vi "VI Anlagengrenzwerte.vi"() -> ()   [LabVIEW 2020, in "Anlagengrenzwerte.lvlib"]
uses:
  Seiten/Anlagengrenzwerte/Anlagengrenzwerte.lvlib
  Visualisierungs Elemente/Button.ctl
  Seiten/Anlagengrenzwerte/Anlagen-Grenzwerte Anzeige.ctl
  Seiten/Anlagengrenzwerte/Anlagen-Parameter Anzeige.ctl
  Seiten/Anlagengrenzwerte/FGV Anlagengrenzwerte Aktionen.ctl
  Seiten/Anlagenuebersicht/Aktionen Ausgabefaelder einfaerben.ctl
  Passwortverwaltung/FGV Passwort Aktion.ctl
  Allgemein/Aktionen Daten am cRIO speichern.ctl
  Seiten/FT-IR/FGV FT-IR Diagnose Aktionen.ctl
  Status Analysatoren/Aktion Status Analysatoren.ctl
  Status Analysatoren/Status Analysatoren.lvlib
  Passwortverwaltung/Passwort.lvlib
  Allgemein/allgemeine Sub-VIs.lvlib
  Seiten/Anlagenuebersicht/VisBx Anzeige/Anlagenuebersicht.lvlib
  Seiten/FT-IR/FT-IR.lvlib
  cRIO/PC/Kommunikation mit cRIO.lvlib
  Visualisierungs Elemente/Zahlen-Eingabefeld.ctl
panel:
  out "HL zu FT-IR:":sgl caption="°C" format="%.1f"
  out "Durchfluss CalGas:":sgl caption="l/min" format="%.1f"
  out "Schaltschranktemperatur:":sgl caption="°C" format="%.1f"
  out "Gaskühler:":sgl caption="°C" format="%.1f"
  out "Heizung FT-IR Messzelle:":sgl caption="°C" format="%.1f"
  out "Heizung Extern SP2:":sgl caption="°C" format="%.1f"
  out "Heizung Extern SP1:":sgl caption="°C" format="%.1f"
  out "Heizung Pumpe:":sgl caption="°C" format="%.1f"
  out "Heizung Filter:":sgl caption="°C" format="%.1f"
  out "Druck Kalter Block:":sgl caption="mbar" format="%.1f"
  out "Druck Ausgang:":sgl caption="mbar"
  out "Durchfluss FT-IR:":sgl caption="l/min" format="%.1f"
  out "Eingangsdruck":sgl caption="atm" format="%.3f"
  in  "speichern":T1
  in  "Anlagen-Grenzwerte":T2 {"Heizleitung zu FT-IR:"."Abschalt-Max" format="%#_5g"; "Heizleitung zu FT-IR:"."Abschalt-Min" format="%#_5g"; "Heizleitung zu FT-IR:"."Warn-Max" format="%#_5g"; "Heizleitung zu FT-IR:"."Warn-Min" format="%#_5g"; "Heizleitung zu FT-IR:"."Sollwert" format="%#_5g"; "Heizleitung zu FT-IR:"."Regler" items=["inaktiv", "aktiv"]; "Druck Kalter Block:"."Abschalt-Max" format="%#_5g"; "Druck Kalter Block:"."Abschalt-Min" format="%#_5g"; "Druck Kalter Block:"."Warn-Max" format="%#_5g"; "Druck Kalter Block:"."Warn-Min" format="%#_5g"; "Druck Kalter Block:"."Sollwert" format="%#_5g"; "Druck Kalter Block:"."Regler" items=["inaktiv", "aktiv"]; "Durchfluss CalGas:"."Abschalt-Max" format="%#_5g"; "Durchfluss CalGas:"."Abschalt-Min" format="%#_5g"; "Durchfluss CalGas:"."Warn-Max" format="%#_5g"; "Durchfluss CalGas:"."Warn-Min" format="%#_5g"; "Durchfluss CalGas:"."Sollwert" format="%#_5g"; "Durchfluss CalGas:"."Regler" items=["inaktiv", "aktiv"]; "Heizleitung Extern SP2:"."Abschalt-Max" format="%#_5g"; "Heizleitung Extern SP2:"."Abschalt-Min" format="%#_5g"; "Heizleitung Extern SP2:"."Warn-Max" format="%#_5g"; "Heizleitung Extern SP2:"."Warn-Min" format="%#_5g"; "Heizleitung Extern SP2:"."Sollwert" format="%#_5g"; "Heizleitung Extern SP2:"."Regler" items=["inaktiv", "aktiv"]; "Gaskühler:"."Abschalt-Max" format="%#_5g"; "Gaskühler:"."Abschalt-Min" format="%#_5g"; "Gaskühler:"."Warn-Max" format="%#_5g"; "Gaskühler:"."Warn-Min" format="%#_5g"; "Gaskühler:"."Sollwert" format="%#_5g"; "Gaskühler:"."Regler" items=["inaktiv", "aktiv"]; "Heizleitung Extern SP1:"."Abschalt-Max" format="%#_5g"; "Heizleitung Extern SP1:"."Abschalt-Min" format="%#_5g"; "Heizleitung Extern SP1:"."Warn-Max" format="%#_5g"; "Heizleitung Extern SP1:"."Warn-Min" format="%#_5g"; "Heizleitung Extern SP1:"."Sollwert" format="%#_5g"; "Heizleitung Extern SP1:"."Regler" items=["inaktiv", "aktiv"]; "Schaltschranktemperatur:"."Abschalt-Max" format="%#_5g"; "Schaltschranktemperatur:"."Abschalt-Min" format="%#_5g"; "Schaltschranktemperatur:"."Warn-Max" format="%#_5g"; "Schaltschranktemperatur:"."Warn-Min" format="%#_5g"; "Schaltschranktemperatur:"."Sollwert" format="%#_5g"; "Schaltschranktemperatur:"."Regler" items=["inaktiv", "aktiv"]; "FT-IR Heizung Messzelle:"."Abschalt-Max" format="%#_5g"; "FT-IR Heizung Messzelle:"."Abschalt-Min" format="%#_5g"; "FT-IR Heizung Messzelle:"."Warn-Max" format="%#_5g"; "FT-IR Heizung Messzelle:"."Warn-Min" format="%#_5g"; "FT-IR Heizung Messzelle:"."Sollwert" format="%#_5g"; "FT-IR Heizung Messzelle:"."Regler" items=["inaktiv", "aktiv"]; "Heizung Pumpe:"."Abschalt-Max" format="%#_5g"; "Heizung Pumpe:"."Abschalt-Min" format="%#_5g"; "Heizung Pumpe:"."Warn-Max" format="%#_5g"; "Heizung Pumpe:"."Warn-Min" format="%#_5g"; "Heizung Pumpe:"."Sollwert" format="%#_5g"; "Heizung Pumpe:"."Regler" items=["inaktiv", "aktiv"]; "Heizung Filterblock:"."Abschalt-Max" format="%#_5g"; "Heizung Filterblock:"."Abschalt-Min" format="%#_5g"; "Heizung Filterblock:"."Warn-Max" format="%#_5g"; "Heizung Filterblock:"."Warn-Min" format="%#_5g"; "Heizung Filterblock:"."Sollwert" format="%#_5g"; "Heizung Filterblock:"."Regler" items=["inaktiv", "aktiv"]; "Heizleitungen intern:"."Abschalt-Max" format="%#_5g"; "Heizleitungen intern:"."Abschalt-Min" format="%#_5g"; "Heizleitungen intern:"."Warn-Max" format="%#_5g"; "Heizleitungen intern:"."Warn-Min" format="%#_5g"; "Heizleitungen intern:"."Sollwert" format="%#_5g"; "Heizleitungen intern:"."Regler" items=["inaktiv", "aktiv"]; "Druck Ausgang:"."Abschalt-Max" format="%#_5g"; "Druck Ausgang:"."Abschalt-Min" format="%#_5g"; "Druck Ausgang:"."Warn-Max" format="%#_5g"; "Druck Ausgang:"."Warn-Min" format="%#_5g"; "Druck Ausgang:"."Sollwert" format="%#_5g"; "Druck Ausgang:"."Regler" items=["inaktiv", "aktiv"]; "Durchfluss FT-IR:"."Abschalt-Max" format="%#_5g"; "Durchfluss FT-IR:"."Abschalt-Min" format="%#_5g"; "Durchfluss FT-IR:"."Warn-Max" format="%#_5g"; "Durchfluss FT-IR:"."Warn-Min" format="%#_5g"; "Durchfluss FT-IR:"."Sollwert" format="%#_5g"; "Durchfluss FT-IR:"."Regler" items=["inaktiv", "aktiv"]; "Eingangsdruck FT-IR:"."Abschalt-Max" format="%#_5g"; "Eingangsdruck FT-IR:"."Abschalt-Min" format="%#_5g"; "Eingangsdruck FT-IR:"."Warn-Max" format="%#_5g"; "Eingangsdruck FT-IR:"."Warn-Min" format="%#_5g"; "Eingangsdruck FT-IR:"."Sollwert" format="%#_5g"; "Eingangsdruck FT-IR:"."Regler" items=["inaktiv", "aktiv"]}
  # "Anlagengrenzwerte"
  # "Warngrenzen"
  # "Abschaltgrenzen"
  # "Regelung\naktiv/inaktiv"
  # "Parameter"
  # "Actual value"
  # "Sollwert"
  # "Min"
  # "Max"
  # "Min"
  # "Max"
  # "°C"
  # "°C"
  # "°C"
  # "mbar"
  # "mbar"
  # "mbar"
  # "l/min"
  # "l/min"
  # "l/min"
  # "°C"
  # "°C"
  # "°C"
  # "°C"
  # "°C"
  # "°C"
  # "°C"
  # "°C"
  # "°C"
  # "°C"
  # "°C"
  # "°C"
  # "°C"
  # "°C"
  # "°C"
  # "°C"
  # "°C"
  # "°C"
  # "°C"
  # "°C"
  # "°C"
  # "°C"
  # "°C"
  # "°C"
  # "mbar"
  # "mbar"
  # "mbar"
  # "l/min"
  # "l/min"
  # "l/min"
  # "atm"
  # "atm"
  # "atm"
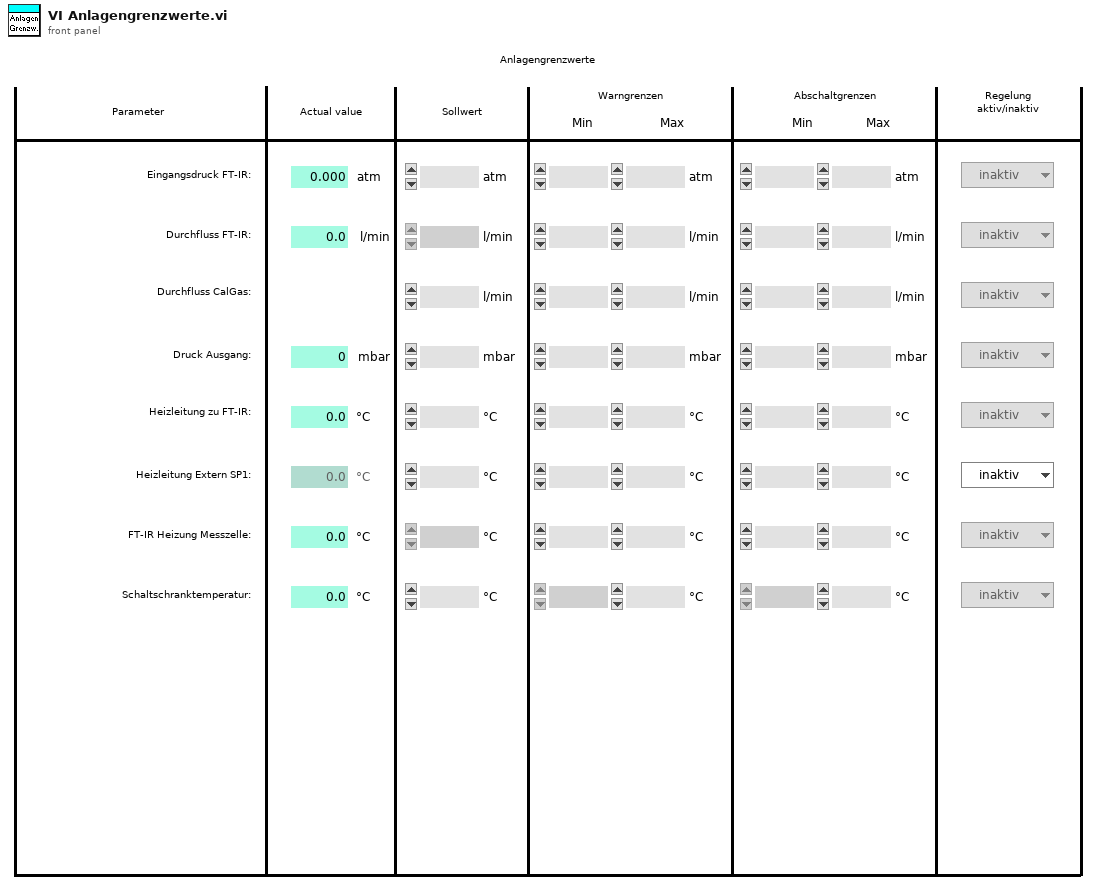
[diagram p1: front panel]
types:
  T1 = typedef "Button.ctl" = bool
  T2 = typedef "Anlagengrenzwerte.lvlib/Anlagen-Grenzwerte Anzeige.ctl" = cluster{"Eingangsdruck FT-IR:":T3, "Durchfluss FT-IR:":T3, "Durchfluss CalGas:":T3, "Druck Ausgang:":T3, "Druck Kalter Block:":T3, "Heizleitungen intern:":T3, "Heizleitung zu FT-IR:":T3, "Heizung Filterblock:":T3, "Heizung Pumpe:":T3, "Heizleitung Extern SP1:":T3, "Heizleitung Extern SP2:":T3, "FT-IR Heizung Messzelle:":T3, "Schaltschranktemperatur:":T3, "Gaskühler:":T3}
  T3 = typedef "Anlagengrenzwerte.lvlib/Anlagen-Parameter Anzeige.ctl" = cluster{"Sollwert":sgl, "Warn-Min":sgl, "Warn-Max":sgl, "Abschalt-Min":sgl, "Abschalt-Max":sgl, "Regler":u16}
  T4 = typedef "Anlagengrenzwerte.lvlib/FGV Anlagengrenzwerte Aktionen.ctl" = enum16{"Lesen", "Grenzwerte schreiben"}
  T5 = typedef "Anlagenuebersicht.lvlib/Aktionen Ausgabefaelder einfaerben.ctl" = enum16{"lesen", "prüfen", "initialisieren"}
  T6 = typedef "Zahlen-Eingabefeld.ctl" = sgl
  T7 = enum8{"Enabled", "Disabled", "Disabled and Grayed Out"}
  T8 = typedef "Passwort.lvlib/FGV Passwort Aktion.ctl" = enum16{"prüfen", "setzen", "Initialisieren", "PW speichern", "lesen", "PW Änderung"}
  T9 = typedef "Status Analysatoren.lvlib/Aktion Status Analysatoren.ctl" = enum16{"lesen", "initialisieren", "Analysatoren aktiv", "FTIR Fehler", "FID Fehler", "PMA Fehler", "Felder einfärben"}
  T10 = typedef "allgemeine Sub-VIs.lvlib/Aktionen Daten am cRIO speichern.ctl" = enum16{"lesen", "speichern setzen", "speichern reset", "gespeichert"}
  T11 = typedef "FT-IR.lvlib/FGV FT-IR Diagnose Aktionen.ctl" = enum16{"Lesen", "Diagnose Schreiben", "Min Schreiben", "Max Schreiben"}
  T12 = typedef "Status Analysatoren.lvlib/Status.ctl" = cluster{"FT-IR aktiv":bool, "FT-IR Fehler":bool, "FID aktiv":bool, "FID Fehler":bool, "PMA aktiv":bool, "PMA Fehler":bool}
  T13 = typedef "Zahlen-Ausgabefeld.ctl" = sgl
  T14 = typedef "Verwaltung - cRIO.lvlib/Analog Eingaenge.ctl" = cluster{"AI0: Durchfluss FT-IR":sgl, "AI1: Druck Ausgang":sgl, "AI2: Umgebungsdruck":sgl, "AI3: Druck FT-IR":sgl, "AI4: Druck CalGas":sgl, "AI5: Reserve":sgl, "AI6: Reserve":sgl, "AI7: Reserve":sgl, "Rohwert Durchfluss FT-IR":sgl, "Rohwert Druck Ausgang":sgl, "Rohwert Umgebungsdruck":sgl, "Rohwert Druck FT-IR":sgl, "Rohwert Druck CalGas":sgl, "Rohwert AI5":sgl, "Rohwert AI6":sgl, "Rohwert AI7":sgl, "Rohwert Diffdruck mbar FTIR":sgl}
  T15 = typedef "Verwaltung - cRIO.lvlib/TC Eingaenge.ctl" = cluster{"TC0: Reserve":sgl, "TC1: HL zu FT-IR":sgl, "TC2: HL Extern SP1":sgl, "TC3: HL Extern SP2":sgl, "TC4: Reserve":sgl, "TC5: Reserve":sgl, "TC6: Reserve":sgl, "TC7: Reserve":sgl, "TC8: FT-IR":sgl, "TC9: Reserve":sgl, "TC10: Schaltschrank":sgl, "TC11: Umgebung":sgl}
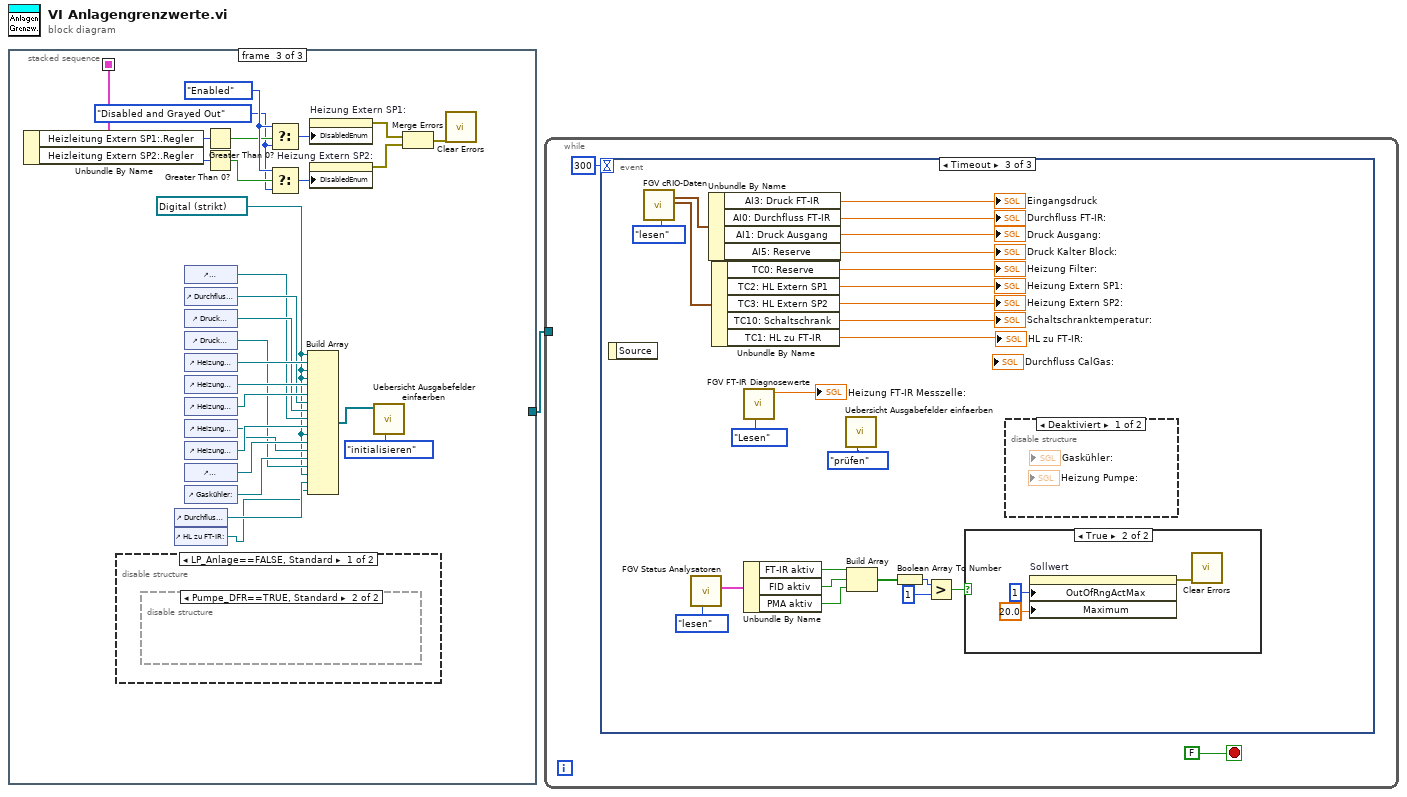
[diagram p0: block diagram]
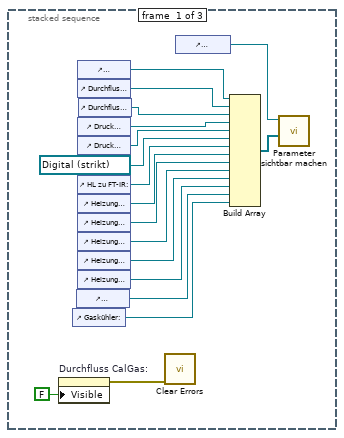
[diagram p2: hidden frame]
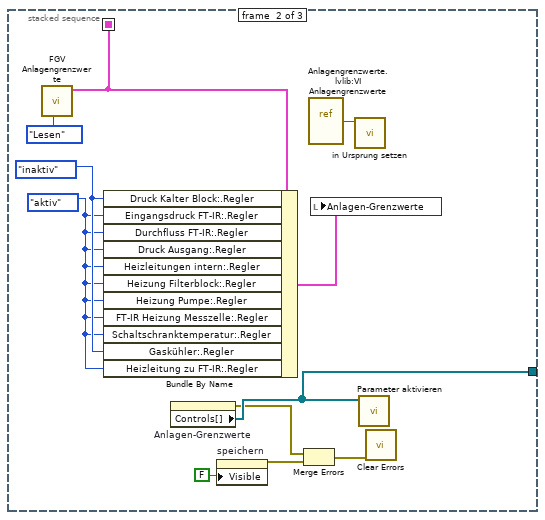
[diagram p3: hidden frame]
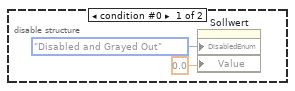
[diagram p4: hidden frame]
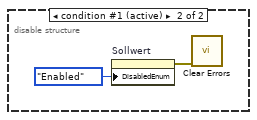
[diagram p5: hidden frame]
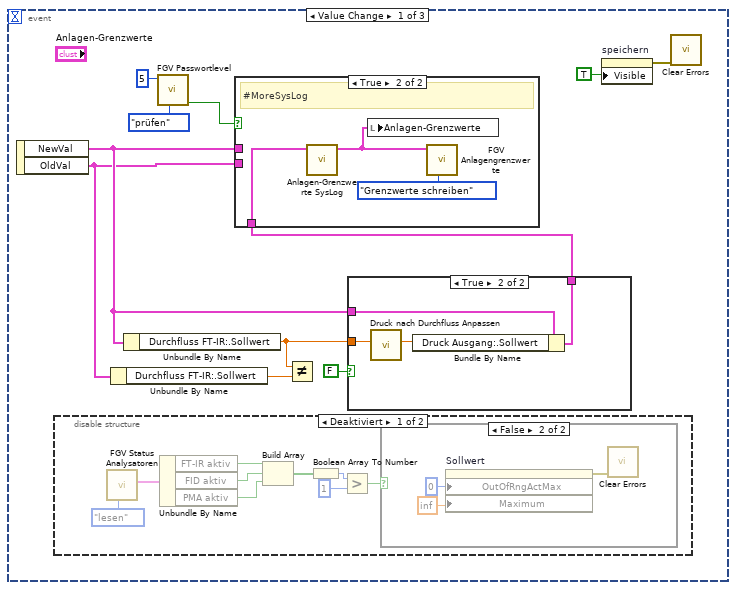
[diagram p6: hidden frame]
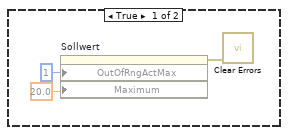
[diagram p7: hidden frame]
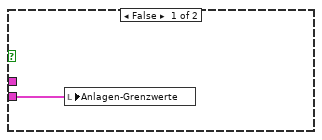
[diagram p10: hidden frame]
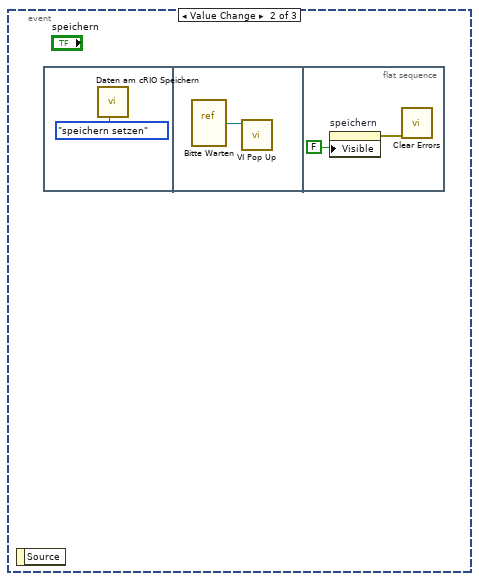
[diagram p11: hidden frame]
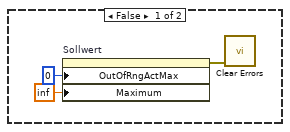
[diagram p13: hidden frame]
diagram:
  n1 = stacked-sequence {
    seq-local: [_ w22 _] -> [_ _ w54]
    tunnel: [_ w29 _] -> w1
    frame #0 {
      n2 = property on="Durchfluss CalGas:" class="DigWert (strikt)"("Visible"=FALSE ("Sichtbar")) -> (error out=w2:errorcluster)  [unwired: 2 in, 1 out]
      n3 = control-ref of="Gaskühler:"() -> (w5:refnum<vi>)
      n4 = control-ref of="Schaltschranktemperatur:"() -> (w6:refnum<vi>)
      n5 = control-ref of="Eingangsdruck"() -> (w10:refnum<vi>)
      n6 = control-ref of="Durchfluss FT-IR:"() -> (w11:refnum<vi>)
      n7 = control-ref of="Druck Ausgang:"() -> (w12:refnum<vi>)
      n8 = control-ref of="Druck Kalter Block:"() -> (w13:refnum<vi>)
      n9 = control-ref of="HL zu FT-IR:"() -> (w8:refnum<vi>)
      n10 = control-ref of="Heizung Filter:"() -> (w7:refnum<vi>)
      n11 = control-ref of="Heizung Pumpe:"() -> (w15:refnum<vi>)
      n12 = control-ref of="Heizung Extern SP1:"() -> (w16:refnum<vi>)
      n13 = control-ref of="Heizung Extern SP2:"() -> (w17:refnum<vi>)
      n14 = control-ref of="Heizung FT-IR Messzelle:"() -> (w18:refnum<vi>)
      n15 = control-ref of="Durchfluss CalGas:"() -> (w4:refnum<vi>)
      n16 = call <vilib>:"Clear Errors.vi"("error in (no error)"=w2) -> ()  [unwired: 5 in, 2 out]
      n17 = control-ref of="Anlagen-Grenzwerte"() -> (w9:refnum<vi>)
      n18 = Build Array(w10, w11, w4, w12, w13, refnum<vi> refnum ("Eingangsdruck"), w8, w7, w15, w16, w17, w18, w6, w5) -> (w19:refnum<vi>[])
      n19 = call "Parameter sichtbar machen.vi"("Istwert Ref"=w19, "Anlagen-Grenzwerte"=w9) -> ()  [unwired: 9 in, 1 out]
    }
    frame #1 {
      w21 = enum16{"inaktiv", "aktiv"}."inaktiv" ("Durchfluss FT-IR:.Regler")
      w20 = enum16{"inaktiv", "aktiv"}."aktiv" ("Durchfluss FT-IR:.Regler")
      n20 = call "FGV Anlagengrenzwerte.vi"("Aktion"=FGV_Anlagengrenzwerte_Aktionen."Lesen") -> ("Anlagen-Grenzwerte Anzeige"=w22:T2)  [unwired: 1 in, 9 out]
      n21 = Bundle By Name(cluster=w22, "Druck Kalter Block:.Regler"=w21, "Eingangsdruck FT-IR:.Regler"=w20, "Durchfluss FT-IR:.Regler"=w20, "Druck Ausgang:.Regler"=w20, "Heizleitungen intern:.Regler"=w20, "Heizung Filterblock:.Regler"=w20, "Heizung Pumpe:.Regler"=w20, "FT-IR Heizung Messzelle:.Regler"=w20, "Schaltschranktemperatur:.Regler"=w20, "Gaskühler:.Regler"=w21, "Heizleitung zu FT-IR:.Regler"=w20) -> (w27:T2)
      n22 = property on="Anlagen-Grenzwerte" class="Cluster (strikt)"() -> (error out=w25:errorcluster, "Controls[]"=w29:refnum<vi>[])  [unwired: 2 in, 1 out]
      n23 = property on="speichern" class="Bool."("Visible"=FALSE ("Sichtbar")) -> (error out=w26:errorcluster)  [unwired: 2 in, 1 out]
      n24 = Merge Errors(w25, w26) -> (w24:errorcluster)
      n25 = vi-ref "Anlagengrenzwerte.lvlib:VI Anlagengrenzwerte.vi"() -> (w23:refnum<vi>)
      n26 = local write "Anlagen-Grenzwerte"(w27) -> ()
      n27 = call "in Ursprung setzen.vi"("VI Referenz"=w23) -> ()  [unwired: 10 in, 1 out]
      n28 = call "Parameter aktivieren.vi"("Ref Anzeige"=w29) -> ()  [unwired: 11 out]
      n29 = call <vilib>:"Clear Errors.vi"("error in (no error)"=w24) -> ()  [unwired: 5 in, 2 out]
    }
    frame #2 {
      w48 = T7."Disabled and Grayed Out" ("Deaktiviert")
      w50 = T7."Enabled" ("Deaktiviert")
      w34 = refnum<vi> refnum ("Eingangsdruck")
      n30 = Unbundle By Name(w54) -> ("Heizleitung Extern SP1:.Regler"=w53:u16, "Heizleitung Extern SP2:.Regler"=w52:u16)
      n31 = disable-structure shown="LP_Anlage==FALSE, Standard" {
        frame condition #0 {
          n32 = disable-structure shown="Pumpe_DFR==TRUE, Standard" {
            frame condition #0 {
              n33 = property on="Sollwert" class="DigWert (strikt)"("DisabledEnum"=T7."Disabled and Grayed Out" ("Deaktiviert"), "Value"=T6 0.0 ("Wert")) -> ()  [unwired: 2 in, 2 out]
            }
            frame condition #1 (active) {
            }
          }
        }
        frame condition #1 (active) {
          n34 = property on="Sollwert" class="DigWert (strikt)"("DisabledEnum"=T7."Enabled" ("Deaktiviert")) -> (error out=w61:errorcluster)  [unwired: 2 in, 1 out]
          n35 = call <vilib>:"Clear Errors.vi"("error in (no error)"=w61) -> ()  [unwired: 5 in, 2 out]
        }
      }
      n36 = control-ref of="Durchfluss CalGas:"() -> (w32:refnum<vi>)
      n37 = control-ref of="HL zu FT-IR:"() -> (w31:refnum<vi>)
      n38 = control-ref of="Eingangsdruck"() -> (w40:refnum<vi>)
      n39 = control-ref of="Durchfluss FT-IR:"() -> (w42:refnum<vi>)
      n40 = control-ref of="Druck Ausgang:"() -> (w41:refnum<vi>)
      n41 = control-ref of="Druck Kalter Block:"() -> (w35:refnum<vi>)
      n42 = control-ref of="Heizung Filter:"() -> (w45:refnum<vi>)
      n43 = control-ref of="Heizung Pumpe:"() -> (w44:refnum<vi>)
      n44 = control-ref of="Heizung Extern SP1:"() -> (w43:refnum<vi>)
      n45 = control-ref of="Heizung Extern SP2:"() -> (w37:refnum<vi>)
      n46 = control-ref of="Heizung FT-IR Messzelle:"() -> (w39:refnum<vi>)
      n47 = control-ref of="Schaltschranktemperatur:"() -> (w38:refnum<vi>)
      n48 = control-ref of="Gaskühler:"() -> (w36:refnum<vi>)
      n49 = Greater Than 0?(x=w53) -> (x > 0?=w49:bool)
      n50 = Greater Than 0?(x=w52) -> (x > 0?=w51:bool)
      n51 = Select(t=w50, s=w49, f=w48) -> (s? t:f=w47:T7)
      n52 = Select(t=w50, s=w51, f=w48) -> (s? t:f=w46:T7)
      n53 = Build Array(w34, w45, w34, w34, w44, w43, w42, w41, w40, w39, w34, w38, w37, w36, w35, w34, w32, w31) -> (w33:refnum<vi>[])
      n54 = property on="Heizung Extern SP1:" class="DigWert (strikt)"("DisabledEnum"=w47) -> (error out=w57:errorcluster)  [unwired: 2 in, 1 out]
      n55 = property on="Heizung Extern SP2:" class="DigWert (strikt)"("DisabledEnum"=w46) -> (error out=w56:errorcluster)  [unwired: 2 in, 1 out]
      n56 = call "Uebersicht Ausgabefelder einfaerben.vi"("Aktionen"=Aktionen_Ausgabefaelder_einfaerben."initialisieren", "Angehängtes Array"=w33) -> ()  [unwired: 10 in]
      n57 = Merge Errors(w57, w56) -> (w55:errorcluster)
      n58 = call <vilib>:"Clear Errors.vi"("error in (no error)"=w55) -> ()  [unwired: 5 in, 2 out]
    }
  }
  n59 = while {
    tunnel: w1 -> [_]
    stop <- FALSE stop-if-true
    n60 = event shown="[2] Timeout" {
      selector: _ -> [_ _ _]
      dyn-events: _ -> [_ _ _]
      timeout: 300 -> [_ _ _]
      event Value Change {
        n61 = event-data() -> ("NewVal"=w68:T2, "OldVal"=w66:T2)  [unwired: 1 out]
        n62 = disable-structure shown="Deaktiviert" {
          frame Disabled {
            n63 = call "FGV Status Analysatoren.vi"("Aktionen"=Aktion_Status_Analysatoren."lesen") -> ("Status Analysatoren"=w83:T12)  [unwired: 10 in]
            n64 = Unbundle By Name(w83) -> ("FT-IR aktiv"=w82:bool, "FID aktiv"=w81:bool, "PMA aktiv"=w80:bool)
            n65 = Build Array(w82, w81, w80) -> (w79:bool[])
            n66 = Boolean Array To Number(Boolean array=w79) -> (number=w78:u32)
            n67 = Greater?(x=w78, y=u32 1) -> (0:w76:bool)
            n68 = case shown="False" w76 {
              frame True {
                n69 = property on="Sollwert" class="DigWert (strikt)"("OutOfRngActMax"=u8 1 ("Werte außerhalb der Grenzen:Maximum"), "Maximum"=20.0 ("Wertebereich:Maximum")) -> (error out=w85:errorcluster)  [unwired: 2 in, 1 out]
                n70 = call <vilib>:"Clear Errors.vi"("error in (no error)"=w85) -> ()  [unwired: 5 in, 2 out]
              }
              frame False {
                n71 = property on="Sollwert" class="DigWert (strikt)"("OutOfRngActMax"=u8 0 ("Werte außerhalb der Grenzen:Maximum"), "Maximum"=inf ("Wertebereich:Maximum")) -> (error out=w88:errorcluster)  [unwired: 2 in, 1 out]
                n72 = call <vilib>:"Clear Errors.vi"("error in (no error)"=w88) -> ()  [unwired: 5 in, 2 out]
              }
            }
          }
          frame Enabled {
          }
        }
        n73 = Unbundle By Name(w66) -> ("Durchfluss FT-IR:.Sollwert"=w70:sgl)
        n74 = Unbundle By Name(w68) -> ("Durchfluss FT-IR:.Sollwert"=w69:sgl)
        n75 = call "FGV Passwortlevel.vi"("FGV Passwort Aktion"=FGV_Passwort_Aktion."prüfen", "geforderter Level"=i16 5) -> ("Freigabe"=w72:bool)  [unwired: 2 in, 7 out]
        n76 = Not Equal?(x=w69, y=w70) -> ()  [unwired: 1 out]
        n77 = case shown="True" FALSE {
          tunnel: w69 -> [_ w95]
          tunnel: w68 -> [w91 w93]
          tunnel: [w91 w92] -> w67
          frame False {
            # "DEAKTIVIERT wegen PMD"
          }
          frame True {
            n78 = call "Druck nach Durchfluss Anpassen.vi"("Sollwert Durchfluss"=w95) -> ("Druck Ausgang"=w94:T13)  [unwired: 10 in]
            n79 = Bundle By Name(cluster=w93, "Druck Ausgang:.Sollwert"=w94) -> (w92:T2)
          }
        }
        n80 = case shown="True" w72 {
          tunnel: w68 -> [_ _]
          tunnel: w66 -> [w96 _]
          tunnel: w67 -> [_ w98]
          frame False {
            n81 = local write "Anlagen-Grenzwerte"(w96) -> ()
          }
          frame True {
            # "#MoreSysLog"
            n82 = call "Anlagen-Grenzwerte SysLog.vi"("NewVal"=w98) -> ("NewVal out"=w97:T2)  [unwired: 10 in]
            n83 = local write "Anlagen-Grenzwerte"(w97) -> ()
            n84 = call "FGV Anlagengrenzwerte.vi"("Aktion"=FGV_Anlagengrenzwerte_Aktionen."Grenzwerte schreiben", "Anlagen-Grenzwerte Anzeige"=w97) -> ()  [unwired: 10 out]
          }
        }
        n85 = property on="speichern" class="Bool."("Visible"=TRUE ("Sichtbar")) -> (error out=w71:errorcluster)  [unwired: 2 in, 1 out]
        n86 = call <vilib>:"Clear Errors.vi"("error in (no error)"=w71) -> ()  [unwired: 5 in, 2 out]
      }
      event Value Change {
        n87 = event-data() -> ()  [unwired: 2 out]
        n88 = flat-sequence {
          frame #0 {
            n89 = call "Daten am cRIO Speichern.vi"("Aktionen"=Aktionen_Daten_am_cRIO_speichern."speichern setzen") -> ()  [unwired: 9 in, 2 out]
          }
          frame #1 {
            n90 = vi-ref "Bitte Warten.vi"() -> (w101:refnum<vi>)
            n91 = call "VI Pop Up.vi"("VI Referenz"=w101) -> ()  [unwired: 10 in, 1 out]
          }
          frame #2 {
            n92 = property on="speichern" class="Bool."("Visible"=FALSE ("Sichtbar")) -> (error out=w102:errorcluster)  [unwired: 2 in, 1 out]
            n93 = call <vilib>:"Clear Errors.vi"("error in (no error)"=w102) -> ()  [unwired: 5 in, 2 out]
          }
        }
      }
      event Timeout {
        n94 = event-data() -> ()  [unwired: 2 out]
        n95 = call "FGV cRIO-Daten.vi"("Aktion"=enum16{"lesen", "schreiben"}."lesen") -> ("Analog Input"=w126:T14, "TC Eingänge"=w120:T15)  [unwired: 9 in, 8 out]
        n96 = call "FGV Status Analysatoren.vi"("Aktionen"=Aktion_Status_Analysatoren."lesen") -> ("Status Analysatoren"=w112:T12)  [unwired: 10 in]
        n97 = Unbundle By Name(w126) -> ("AI3: Druck FT-IR"=→"Eingangsdruck":sgl, "AI0: Durchfluss FT-IR"=→"Durchfluss FT-IR:":sgl, "AI1: Druck Ausgang"=→"Druck Ausgang:":sgl, "AI5: Reserve"=→"Druck Kalter Block:":sgl)
        n98 = Unbundle By Name(w120) -> ("TC0: Reserve"=→"Heizung Filter:":sgl, "TC2: HL Extern SP1"=→"Heizung Extern SP1:":sgl, "TC3: HL Extern SP2"=→"Heizung Extern SP2:":sgl, "TC10: Schaltschrank"=→"Schaltschranktemperatur:":sgl, "TC1: HL zu FT-IR"=→"HL zu FT-IR:":sgl)
        n99 = call "FGV FT-IR Diagnosewerte.vi"("Aktionen"=FGV_FT-IR_Diagnose_Aktionen."Lesen") -> ("Temperatur"=→"Heizung FT-IR Messzelle:":dbl)  [unwired: 5 in, 5 out]
        n100 = Unbundle By Name(w112) -> ("FT-IR aktiv"=w111:bool, "FID aktiv"=w110:bool, "PMA aktiv"=w109:bool)
        n101 = call "Uebersicht Ausgabefelder einfaerben.vi"("Aktionen"=Aktionen_Ausgabefaelder_einfaerben."prüfen") -> ()  [unwired: 11 in]
        n102 = Build Array(w111, w110, w109) -> (w108:bool[])
        n103 = Boolean Array To Number(Boolean array=w108) -> (number=w107:u32)
        n104 = Greater?(x=w107, y=u32 1) -> (0:w105:bool)
        n105 = case shown="True" w105 {
          frame False {
            n106 = property on="Sollwert" class="DigWert (strikt)"("OutOfRngActMax"=u8 0 ("Werte außerhalb der Grenzen:Maximum"), "Maximum"=inf ("Wertebereich:Maximum")) -> (error out=w129:errorcluster)  [unwired: 2 in, 1 out]
            n107 = call <vilib>:"Clear Errors.vi"("error in (no error)"=w129) -> ()  [unwired: 5 in, 2 out]
          }
          frame True {
            n108 = property on="Sollwert" class="DigWert (strikt)"("OutOfRngActMax"=u8 1 ("Werte außerhalb der Grenzen:Maximum"), "Maximum"=20.0 ("Wertebereich:Maximum")) -> (error out=w131:errorcluster)  [unwired: 2 in, 1 out]
            n109 = call <vilib>:"Clear Errors.vi"("error in (no error)"=w131) -> ()  [unwired: 5 in, 2 out]
          }
        }
        n110 = disable-structure shown="Deaktiviert" {
          frame Disabled {
          }
          frame Enabled {
          }
        }
      }
    }
  }
